vi "UpdateFrontPanel.vi"(8 "ErrorArray In":errorcluster[](array[cluster])) -> (0 "ErrorArray Out":errorcluster[](array[cluster]))   [LabVIEW 2017, in "Framework.lvlib"]
uses:
  Framework.lvlib
  Bus_class/Bus.lvclass
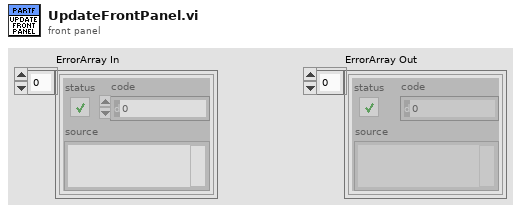
[diagram p1: front panel]
types:
  T1 = typedef "Framework.lvlib/clFrontPanelControlRefs.ctl" = cluster{"TestFilePathRef":refnum<vi>, "BusNumberRef":refnum<vi>, "NumberOfBusesRef":refnum<vi>, "EvtTypeRef":refnum<vi>, "EvtParamsRef":refnum<vi>, "EvtConfigRef":refnum<vi>, "StartTimeRef":refnum<vi>, "EndTimeRef":refnum<vi>, "PmuImpairTypeRef":refnum<vi>, "PmuImpairParamsRef":refnum<vi>, "NetImpairParamsRef":refnum<vi>, "FlagImpairTypeRef":refnum<vi>, "FlagImpairParamsRef":refnum<vi>, "NetImpairTypeRef":refnum<vi>, "OutputFileType":refnum<vi>, "PmuImpairConfigRef":refnum<vi>, "AppTypeRef":refnum<vi>, "ScriptPathRef":refnum<vi>, "ShowPanels?":refnum<vi>}
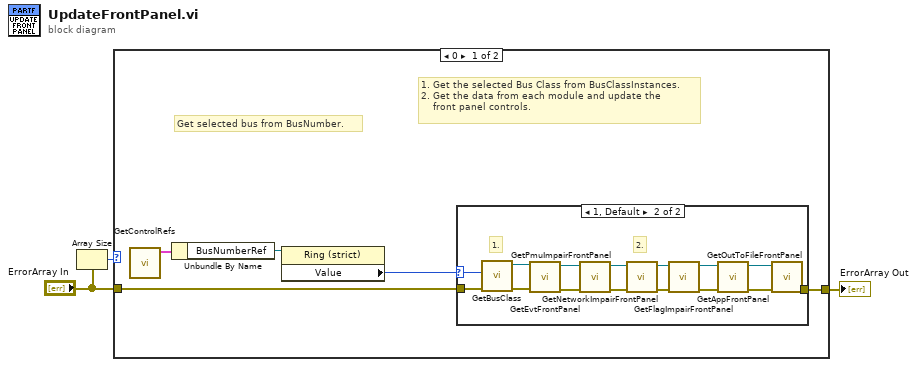
[diagram p0: block diagram]
diagram:
  n1 = Array Size(array="ErrorArray In") -> (size(s)=w3:i32)
  n2 = case shown="0" w3 {
    tunnel: "ErrorArray In" -> [w8 w25]
    tunnel: [w5 w25] -> w1
    frame 0 {
      # "1. Get the selected Bus Class from BusClassInstances.\n2. Get the data from each module and update the\n    front panel controls."
      # "Get selected bus from BusNumber."
      n3 = call "GetControlRefs.vi"() -> ("clControlRefs Out"=w4:T1)  [unwired: 11 in]
      n4 = Unbundle By Name(w4) -> ("BusNumberRef"=w7:refnum<vi>)
      n5 = property class="Ring (strict)"(reference=w7) -> ("Value"=w6:u8)  [unwired: 1 in, 2 out]
      n6 = case shown="1, Default" w6 {
        selector: w6 -> [_ w20]
        tunnel: w8 -> [w9 w24]
        tunnel: [w9 w11] -> w5
        frame 0 {
        }
        frame 1, Default {
          # "2."
          # "1."
          n7 = call "GetBusClass.vi"("ErrorArray In"=w24, "BusNumber"=w20) -> ("ErrorArray Out"=w23:errorcluster[], "Framework.lvlib:Bus.lvclass"=w22:refnum<class "Bus.lvclass">)  [unwired: 8 in]
          n8 = call "GetEvtFrontPanel.vi"("ErrorArray In"=w23, "Bus.lvclass In"=w22) -> ("ErrorArray Out"=w19:errorcluster[], "Bus.lvclass Out"=w21:refnum<class "Bus.lvclass">)  [unwired: 8 in]
          n9 = call "GetPmuImpairFrontPanel.vi"("ErrorArray In"=w19, "Bus.lvclass In"=w21) -> ("ErrorArray Out"=w17:errorcluster[], "Bus.lvclass Out"=w18:refnum<class "Bus.lvclass">)  [unwired: 8 in]
          n10 = call "GetNetworkImpairFrontPanel.vi"("ErrorArray In"=w17, "Bus.lvclass In"=w18) -> ("ErrorArray Out"=w16:errorcluster[], "Bus.lvclass Out"=w15:refnum<class "Bus.lvclass">)  [unwired: 8 in]
          n11 = call "GetFlagImpairFrontPanel.vi"("ErrorArray In"=w16, "Bus.lvclass In"=w15) -> ("ErrorArray Out"=w14:errorcluster[], "Bus.lvclass Out"=w13:refnum<class "Bus.lvclass">)  [unwired: 8 in]
          n12 = call "GetAppFrontPanel.vi"("ErrorArray In"=w14, "Bus.lvclass In"=w13) -> ("ErrorArray Out"=w12:errorcluster[], "Bus.lvclass Out"=w10:refnum<class "Bus.lvclass">)  [unwired: 8 in]
          n13 = call "GetOutToFileFrontPanel.vi"("ErrorArray In"=w12, "Bus.lvclass In"=w10) -> ("ErrorArray Out"=w11:errorcluster[])  [unwired: 8 in, 1 out]
        }
      }
    }
    frame 1, Default {
    }
  }
  "ErrorArray Out" <- w1
